vi "FindMostImportantError.vi"(8 "Errors in":errorcluster[](array[cluster])) -> (0 "error out":errorcluster)   [LabVIEW 2019, in "Tools.lvlib"]
uses:
  Tools.lvlib
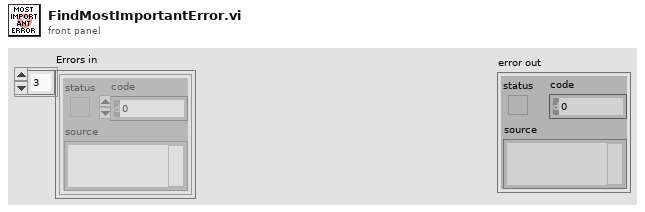
[diagram p1: front panel]
types:
  T1 = cluster{"f":i32, "error in (no error)":errorcluster}
  T2 = cluster{"f":i32, "error in (no error)":errorcluster}[]
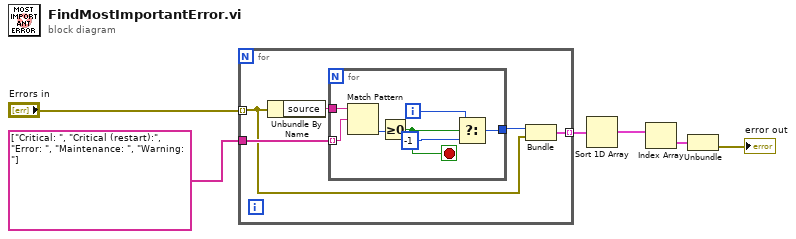
[diagram p0: block diagram]
diagram:
  n1 = for {
    tunnel: "Errors in" -> [w8] mode=indexing
    tunnel: string[] ["Critical: ", "Critical (restart):", "Error: ", "Maintenance: ", "Warning: "] -> [w10]
    tunnel: [w7] -> w4 mode=indexing
    n2 = Unbundle By Name(w8) -> ("source"=w11:string)
    n3 = for {
      tunnel: w11 -> [w18]
      tunnel: w10 -> [w17] mode=indexing
      tunnel: [w12] -> w9
      i -> [w14]
      stop <- w15 stop-if-true
      n4 = Match Pattern(string=w18, regular expression=w17) -> (offset past match=w16:i32)  [unwired: 1 in, 3 out]
      n5 = Greater Or Equal To 0?(x=w16) -> (x >= 0?=w15:bool)
      n6 = Select(t=w14, s=w15, f=-1) -> (s? t:f=w12:i32)
    }
    n7 = Bundle("f"=w9, "error in (no error)"=w8) -> (w7:T1)  [unwired: 1 in]
  }
  n8 = Sort 1D Array(array=w4) -> (sorted array=w3:T2)
  n9 = Index Array(array=w3) -> (element=w2:T1)  [unwired: 1 in]
  n10 = Unbundle(w2) -> ("error in (no error)"=→"error out":errorcluster)  [unwired: 1 out]
